vi "measure_jt.vi"(4 "Skip pixel?":bool, 5 "Date array":string[](array[string]), 6 "Scan settings":T1={"J-V scan"=TRUE, "Start voltage (V)"=0.0, "End voltage (V)"=0.0, "Step voltage (V)"=1.4, "Scan both directions"=TRUE, "Inverted device structure"=FALSE, "Measurement delay (s)"=10.0, "Measurement speed"=0, "Scan rate (V/s)"=0.0, "Stabilisation time (s)"=0.0, "Stabilisation mode"=0, "Stabilisation value (V or A) "=1.0, "Illumination"=0, "Stabilisation in the dark?"=FALSE, "Repeat light scans"=FALSE, "No. of repeat scans"=0.0, "Only repeat for best pixel"=1, "J-t scan"=FALSE, "J-t best pixel only"=7, "J-t start voltage (V)"=0.0, "J-t end voltage (V)"=1.4, "J-t step voltage (V)"=0.01, "Step time (s)"=0.7, "J-t scan both directions"=TRUE, "J-t inverted device structure"=FALSE, "Settling delay (s)"=0.0, "J-t measurement speed"=0, "J-t illumination"=2, "Max. power stabilisation"=FALSE, "Max power best pixel only"=1, "Max. power point tracker"=FALSE, "Vmp from J-V scan"=FALSE, "Max P stab. Specific voltage"=FALSE, "Vmp (V)"=1.0, "Stabilisation time step (s)"=1.0, "Total stabilisation time (s)"=100.0} {"Settling delay (s)" min=0.0; "J-t illumination" items=["Light only", "Dark only", "Light then dark", "Dark then light"]; "Measurement speed" items=["Fast", "Normal", "High accuracy"]; "Illumination" items=["Light only", "Dark only", "Light then dark", "Dark then light"]; "Only repeat for best pixel" items=["only for best pixel", "for best 2 pixels", "for best 3 pixels", "for best 4 pixels", "for best 5 pixels", "for best 6 pixels", "for best 7 pixels", "for all pixels"]; "No. of repeat scans" min=1.0 step=1.0; "Max power best pixel only" items=["only the best pixel", "the best 2 pixels", "the best 3 pixels", "the best 4 pixels", "the best 5 pixels", "the best 6 pixels", "the best 7 pixels", "all pixels"]; "J-t best pixel only" items=["only the best pixel", "the best 2 pixels", "the best 3 pixels", "the best 4 pixels", "the best 5 pixels", "the best 6 pixels", "the best 7 pixels", "all pixels"]; "J-t measurement speed" items=["Fast", "Normal", "High Accuracy"]; "Stabilisation mode" items=["V", "I"]; "Measurement delay (s)" min=0.01}, 7 "Cell details cluster":T2={"Cell Position"=16, "Cell Label"="", "Pixel to measure"=0, "Area (cm^2)"=0.126, "Variable"="", "Variable value"="", "Scan settings in queue"=0, "Light or dark"="", "Measurement Type"=""} {"Pixel to measure" items=["All", "1", "2", "3", "4", "5", "6", "7", "8"]}, 8 "VISA resource name":refnum<visa-resource-name>="GPIB1::24::INSTR", 9 "Intensity (no. of suns)":string, 10 "Experiment Title":string, 11 "User Name":string) -> (3 "Jt Curve":cluster{"Y":dbl[], "Y":dbl[]}[](graph) caption="JV Curve")   [LabVIEW 2016]
uses:
  TypeDefs/scan_settings.ctl
  <vilib>/Utility/file.llb/Read Delimited Spreadsheet (DBL).vi
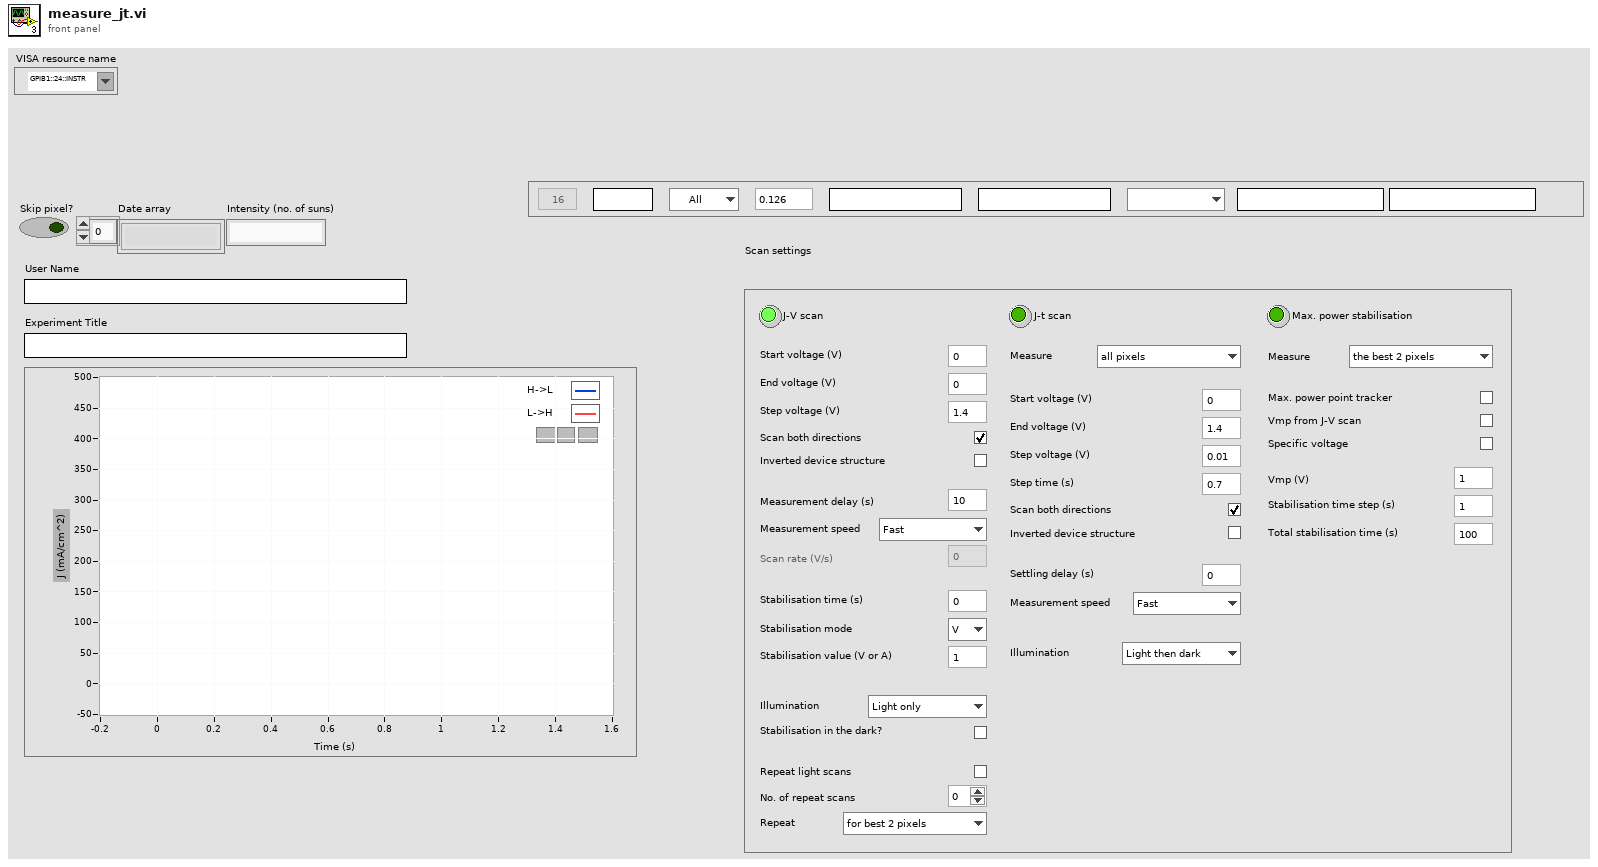
[diagram p1: front panel]
types:
  T1 = typedef "scan_settings.ctl" = cluster{"J-V scan":bool, "Start voltage (V)":dbl, "End voltage (V)":dbl, "Step voltage (V)":dbl, "Scan both directions":bool, "Inverted device structure":bool, "Measurement delay (s)":dbl, "Measurement speed":u8, "Scan rate (V/s)":dbl, "Stabilisation time (s)":dbl, "Stabilisation mode":u16, "Stabilisation value (V or A) ":dbl, "Illumination":u16, "Stabilisation in the dark?":bool, "Repeat light scans":bool, "No. of repeat scans":dbl, "Only repeat for best pixel":u16, "J-t scan":bool, "J-t best pixel only":u16, "J-t start voltage (V)":dbl, "J-t end voltage (V)":dbl, "J-t step voltage (V)":dbl, "Step time (s)":dbl, "J-t scan both directions":bool, "J-t inverted device structure":bool, "Settling delay (s)":dbl, "J-t measurement speed":u16, "J-t illumination":u16, "Max. power stabilisation":bool, "Max power best pixel only":u16, "Max. power point tracker":bool, "Vmp from J-V scan":bool, "Max P stab. Specific voltage":bool, "Vmp (V)":dbl, "Stabilisation time step (s)":dbl, "Total stabilisation time (s)":dbl}
  T2 = cluster{"Cell Position":i32, "Cell Label":string, "Pixel to measure":u16, "Area (cm^2)":dbl, "Variable":string, "Variable value":string, "Scan settings in queue":u16, "Light or dark":string, "Measurement Type":string}
  T3 = typedef "imagedata.ctl" = cluster{"image type":i32, "image depth":i32, "image":u8[], "mask":u8[], "colors":u32[], "Rectangle":cluster{"left":i16, "top":i16, "right":i16, "bottom":i16}}
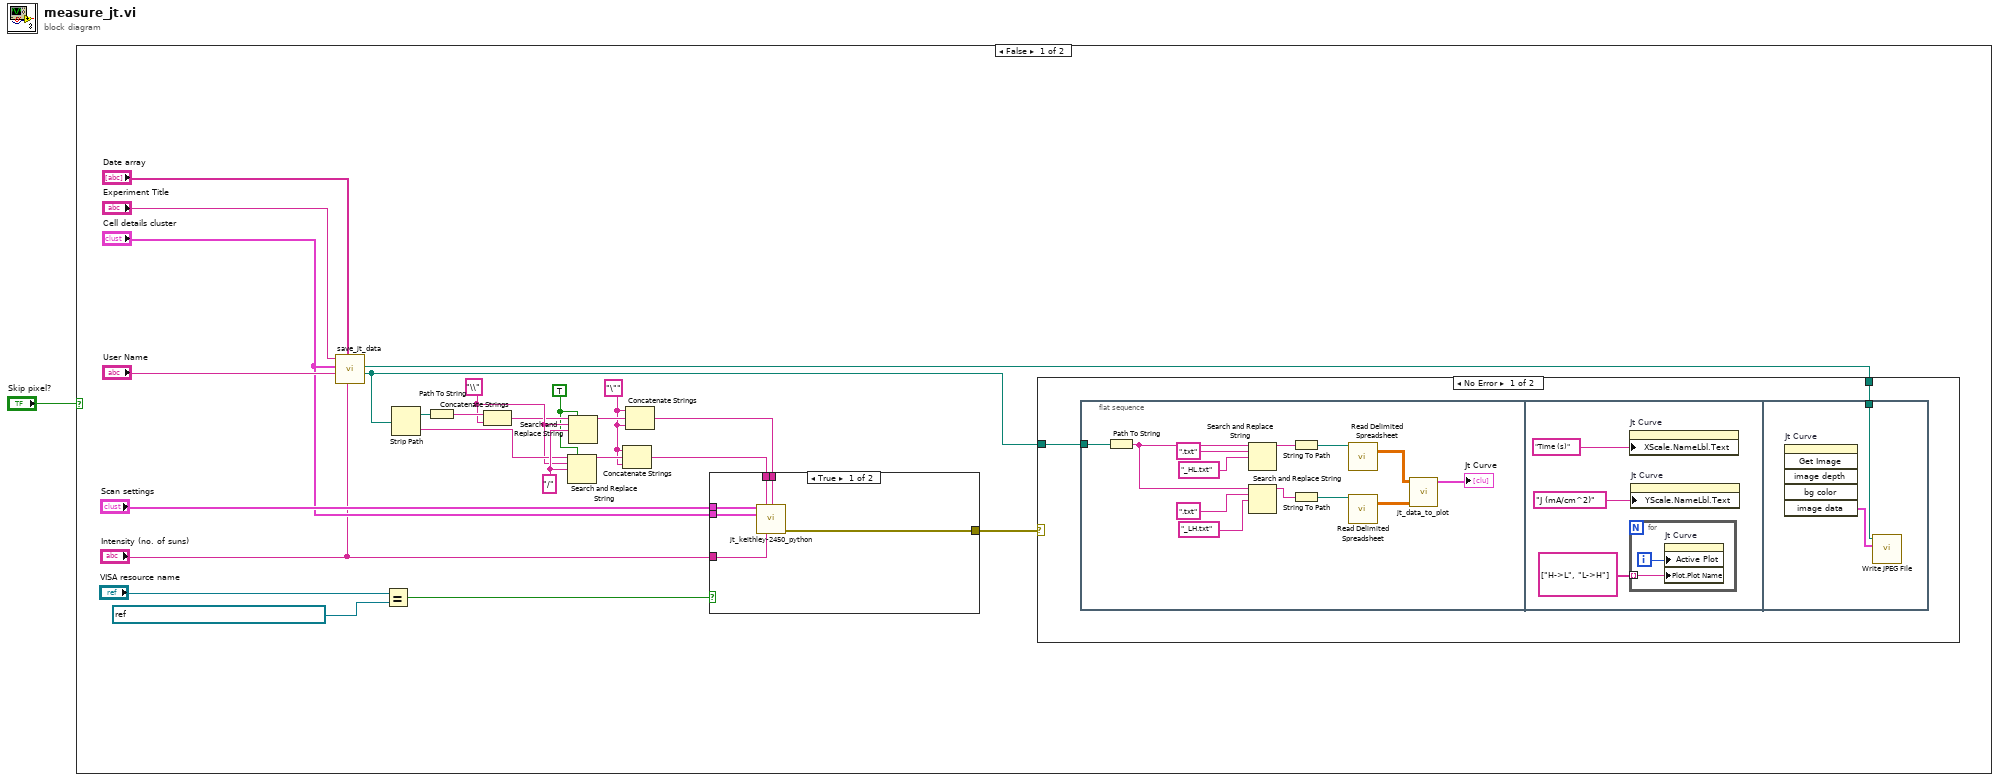
[diagram p0: block diagram]
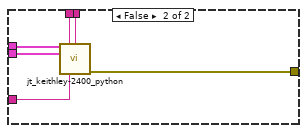
[diagram p3: hidden frame]
diagram:
  n1 = case shown="False" "Skip pixel?" {
    frame False {
      w16 = "\"" ("string")
      w13 = TRUE ("replace all? (F)")
      w21 = "/" ("search string")
      w15 = "\\" ("search string")
      n2 = call "save_jt_data.vi"("Intensity (no. of suns)"="Intensity (no. of suns)", "Date array"="Date array", "User name"="User Name", "Cell details cluster"="Cell details cluster", "Experiment title"="Experiment Title") -> ("File path for JV data"=w7:path, "File path for JV image"=w6:path)  [unwired: 3 in]
      n3 = Equal?(x="VISA resource name", y=refnum<visa-resource-name> "USB0::0x05E6::0x2450::04049675::INSTR") -> (x = y?=w2:bool)
      n4 = Strip Path(path=w7) -> (stripped path=w18:path, name=w19:string)
      n5 = Path To String(path=w18) -> (string=w17:string)
      n6 = Concatenate Strings(w17, w15) -> (w14:string)
      n7 = Search and Replace String(replace all?=w13, input string=w19, search string=w15, replace string=w21) -> (result string=w20:string)  [unwired: 4 in, 3 out]
      n8 = Search and Replace String(replace all?=w13, input string=w14, search string=w15, replace string=w21) -> (result string=w22:string)  [unwired: 4 in, 3 out]
      n9 = Concatenate Strings(w16, w20, w16) -> (w11:string)
      n10 = Concatenate Strings(w16, w22, w16) -> (w12:string)
      n11 = case shown="True" w2 {
        tunnel: w12 -> [w51 w59]
        tunnel: w11 -> [w52 w58]
        tunnel: "Scan settings" -> [w53 w57]
        tunnel: "Cell details cluster" -> [w50 w56]
        tunnel: "Intensity (no. of suns)" -> [w49 w55]
        tunnel: [w48 w54] -> w5
        frame True {
          n12 = call "jt_keithley-2450_python.vi"("Scan settings"=w53, "file name"=w52, "folder path"=w51, "Cell details cluster"=w50, "illumination intensity (suns equiv.)"=w49) -> ("error out"=w48:errorcluster)  [unwired: 10 in]
        }
        frame False {
          n13 = call "jt_keithley-2400_python.vi"("Scan settings"=w57, "file name"=w58, "folder path"=w59, "Cell details cluster"=w56, "illumination intensity (suns equiv.)"=w55) -> ("error out"=w54:errorcluster)  [unwired: 10 in]
        }
      }
      n14 = case shown="No Error" w5 {
        tunnel: w7 -> [w27 _]
        tunnel: w6 -> [w26 _]
        frame No Error {
          n15 = flat-sequence {
            tunnel: w27 -> [w39]
            tunnel: w26 -> [w46]
            frame #0 {
              n16 = Path To String(path=w39) -> (string=w35:string)
              n17 = Search and Replace String(input string=w35, search string=".txt", replace string="_HL.txt" ("replace string (\"\")")) -> (result string=w38:string)  [unwired: 5 in, 3 out]
              n18 = Search and Replace String(input string=w35, search string=".txt", replace string="_LH.txt" ("replace string (\"\")")) -> (result string=w30:string)  [unwired: 5 in, 3 out]
              n19 = String To Path(string=w38) -> (path=w37:path)
              n20 = String To Path(string=w30) -> (path=w29:path)
              n21 = call-poly <vilib>:"Read Delimited Spreadsheet.vi"("file path (dialog if empty)"=w37) -> ("all rows"=w36:dbl[][])  [unwired: 9 in, 5 out]
              n22 = call-poly <vilib>:"Read Delimited Spreadsheet.vi"("file path (dialog if empty)"=w29) -> ("all rows"=w28:dbl[][])  [unwired: 9 in, 5 out]
              n23 = call "jt_data_to_plot.vi"("Data Array 2"=w28, "Data Array"=w36) -> ("JV Curve"=→"Jt Curve":cluster{"Y":dbl[], "Y":dbl[]}[])  [unwired: 9 in]
            }
            frame #1 {
              n24 = property on="Jt Curve" class="XYGraph (strict)"("XScale.NameLbl.Text"="Time (s)" ("Y Scale.Name Label.Text")) -> ()  [unwired: 2 in, 2 out]
              n25 = for {
                tunnel: string[] ["H->L", "L->H"] ("Measurement queue") -> [w44] mode=indexing
                i -> [w45]
                n26 = property on="Jt Curve" class="XYGraph (strict)"("Active Plot"=w45, "Plot.Plot Name"=w44) -> ()  [unwired: 2 in, 2 out]
              }
              n27 = property on="Jt Curve" class="XYGraph (strict)"("YScale.NameLbl.Text"="J (mA/cm^2)" ("Y Scale.Name Label.Text")) -> ()  [unwired: 2 in, 2 out]
            }
            frame #2 {
              n28 = invoke on="Jt Curve" class="XYGraph (strict)" method="Get Image"() -> ("image data"=w47:T3)  [unwired: 6 in, 5 out]
              n29 = call <vilib>:"Write JPEG File.vi"("image data"=w47, "path to JPEG file"=w46) -> ()  [unwired: 8 in, 2 out]
            }
          }
        }
        frame Error {
        }
      }
    }
    frame True {
    }
  }
